vi "Build Self Extracting Installer.vi"(10 "Package Version":string="2024.11.5.6") -> (0 "Error Out":errorcluster)   [LabVIEW 2019]
uses:
  <userlib>/LevyLab/Build Support/PostBuildSupport/PostBuildSupport.lvclass
  <vilib>/MakerHub/Toolbox/LMH-Toolbox.lvlib
  <vilib>/AppBuilder/AB_API_Simple/Build Specification Version.ctl
  <vilib>/AppBuilder/AB_API_Simple/NI_App_Builder_API.lvlib
  <vilib>/AppBuilder/AB_API_Simple/Set Build Specification Version (path).vi
  <vilib>/AppBuilder/AB_API_Simple/Build (path).vi
panel:
  in  "Package Source Folder":path=path "C:/user/patrick/git/Multichannel-Lockin/src"
  in  "Output Package File Path":path
  in  "Product Name":string="Multichannel Lockin"
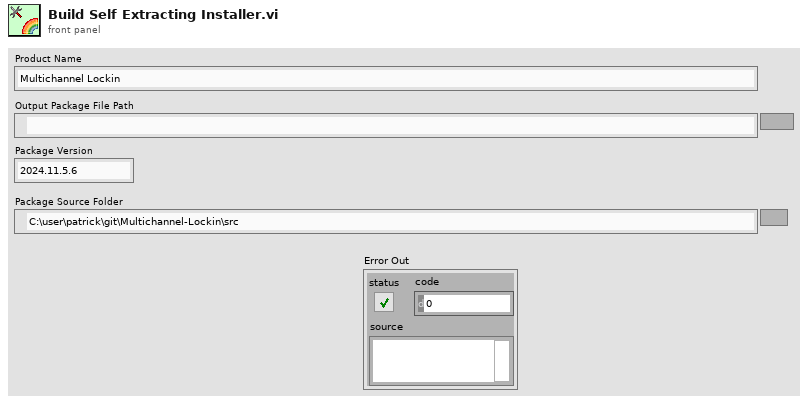
[diagram p1: front panel]
types:
  T1 = typedef "NI_App_Builder_API.lvlib/Build Specification Version.ctl" = cluster{"Major":u16, "Minor":u16, "Fix":u16, "Build":u16}
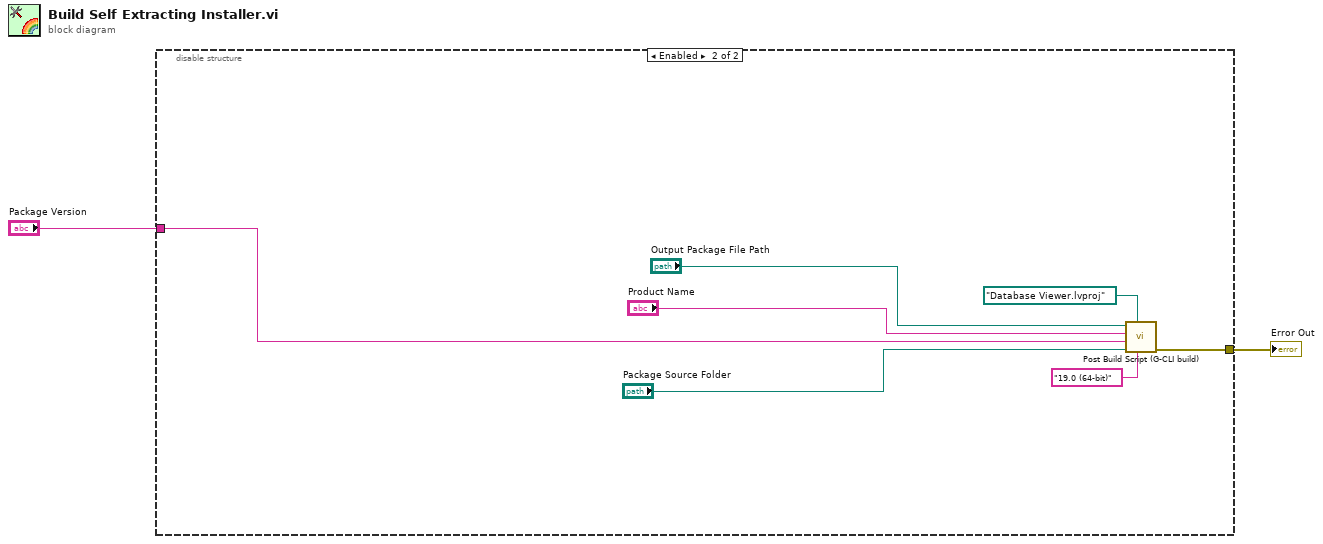
[diagram p0: block diagram]
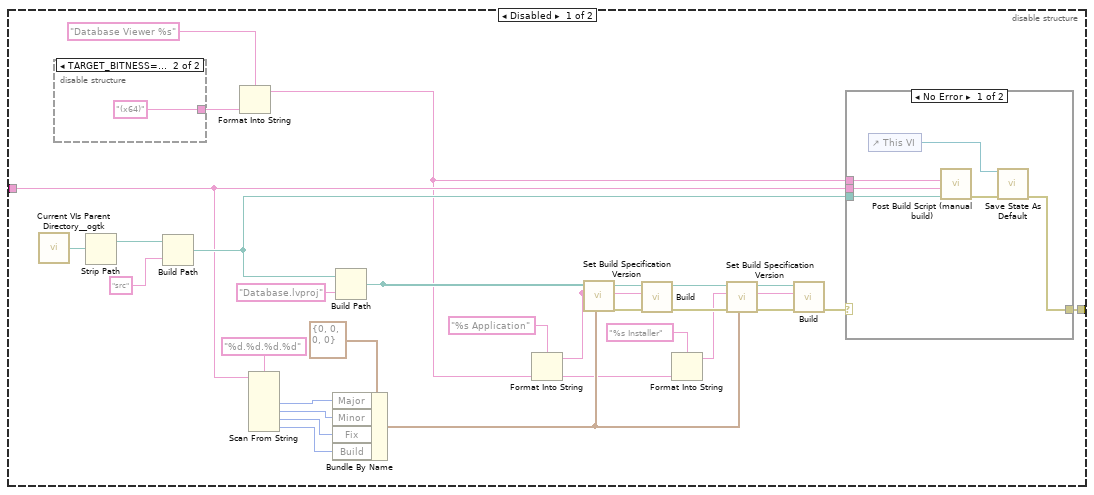
[diagram p2: hidden frame]
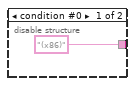
[diagram p3: hidden frame]
diagram:
  n1 = disable-structure shown="Enabled" {
    disable-tunnel: "Package Version" -> [w15 w43]
    disable-tunnel: [w3 w44] -> w1
    frame Disabled {
      n2 = call <userlib>:"Current VIs Parent Directory__ogtk.vi"() -> ("Parent Directory (+ Relative)"=w28:path)  [unwired: 5 in]
      n3 = disable-structure shown="TARGET_BITNESS==64" {
        disable-tunnel: ["(x86)" ("Name of build specification") "(x64)" ("Name of build specification")] -> w6
        frame condition #0 {
        }
        frame condition #1 (active) {
        }
      }
      n4 = Strip Path(path=w28) -> (stripped path=w27:path)  [unwired: 1 out]
      n5 = Build Path(base path=w27, name or relative path="src") -> (appended path=w17:path)
      n6 = Format Into String(format string="Database Viewer %s" ("Product Name"), w6) -> (resulting string=w4:string)  [unwired: 2 in, 1 out]
      n7 = Scan From String(format string="%d.%d.%d.%d", input string=w15) -> (output 1=w22:i32, output 2=w25:i32, output 3=w21:i32, output 4=w24:i32)  [unwired: 6 in, 3 out]
      n8 = Bundle By Name(cluster=T1 {"Major"=0, "Minor"=0, "Fix"=0, "Build"=0} ("Build Specification Version"), "Major"=w22, "Minor"=w25, "Fix"=w21, "Build"=w24) -> (w19:T1)
      n9 = Build Path(base path=w17, name or relative path="Database.lvproj") -> (appended path=w16:path)
      n10 = Format Into String(format string="%s Application" ("Name of build specification"), w4) -> (resulting string=w10:string)  [unwired: 2 in, 1 out]
      n11 = call-poly <vilib>:"Set Build Specification Version.vi"("Build Specification Version"=w19, "Name of build specification"=w10, "Path to project"=w16) -> ("error out"=w14:errorcluster)  [unwired: 8 in]
      n12 = call-poly <vilib>:"Build.vi"("error in (no error)"=w14, "Name of build specification (if empty: build all)"=w10, "Path to project"=w16) -> ("error out"=w13:errorcluster)  [unwired: 7 in, 1 out]
      n13 = Format Into String(format string="%s Installer" ("Name of build specification"), w4) -> (resulting string=w9:string)  [unwired: 2 in, 1 out]
      n14 = call-poly <vilib>:"Set Build Specification Version.vi"("Build Specification Version"=w19, "error in (no error)"=w13, "Name of build specification"=w9, "Path to project"=w16) -> ("error out"=w12:errorcluster)  [unwired: 7 in]
      n15 = call-poly <vilib>:"Build.vi"("error in (no error)"=w12, "Name of build specification (if empty: build all)"=w9, "Path to project"=w16) -> ("error out"=w7:errorcluster)  [unwired: 7 in, 1 out]
      n16 = case shown="No Error" w7 {
        selector: w7 -> [_ w37]
        tunnel: w17 -> [w34 _]
        tunnel: w4 -> [w33 _]
        tunnel: w15 -> [w32 _]
        tunnel: [w31 w37] -> w3
        frame No Error {
          n17 = control-ref of="This VI"() -> (w35:refnum<vi>)
          n18 = call <userlib>:"Post Build Script (manual build).vi"("Package Source Folder"=w34, "Package Version"=w32, "Product Name"=w33) -> ("error out"=w36:errorcluster)  [unwired: 8 in]
          n19 = call <vilib>:"Save State As Default.vi"("Error In"=w36, "Target VI"=w35) -> ("Error Out"=w31:errorcluster)  [unwired: 8 in, 1 out]
        }
        frame Error {
        }
      }
    }
    frame Enabled {
      n20 = call <userlib>:"Post Build Script (G-CLI build).vi"("Package LabVIEW Version (19.0 (32-bit))"="19.0 (64-bit)", "Project File Path"=path "Database Viewer.lvproj", "Package Source Folder"="Package Source Folder", "Package Version (major.minor.patch.build)"=w43, "Product Name"="Product Name", "Output Package File Path"="Output Package File Path") -> ("error out"=w44:errorcluster)  [unwired: 5 in]
    }
  }
  "Error Out" <- w1
